vi "reconnaissance couleur (SubVI).vi"(8 "error in (no error)":errorcluster, 9 "Image Out in":T2, 10 "ROI Descriptor (Color Classification 1)":T1, 11 "Refnum in":T3) -> (1 "Array":errorcluster[](array[cluster]), 2 "Array 2":string[](array[string]), 3 "Refnum out":T2)   [LabVIEW 2019]
uses:
  <vilib>/vision/Image Controls.llb/IMAQ Image.ctl
  <vilib>/vision/Classification.llb/IMAQ Classifier Session.ctl
  <vilib>/vision/NI_Vision_Development_Module.lvlib
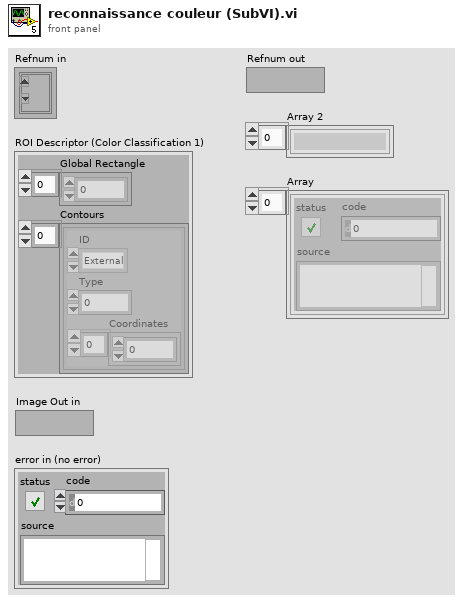
[diagram p1: front panel]
types:
  T1 = cluster{"Global Rectangle":i32[], "Contours":cluster{"ID":enum32{"External", "Internal"}, "Type":u32, "Coordinates":i32[]}[]}
  T2 = typedef "IMAQ Image.ctl" = refnum<image>
  T3 = typedef "IMAQ Classifier Session.ctl" = refnum<k1>
  T4 = typedef "ROI Descriptor" = cluster{"Global Rectangle":i32[], "Contours":cluster{"ID":enum32{"External", "Internal"}, "Type":u32, "Coordinates":i32[]}[]}
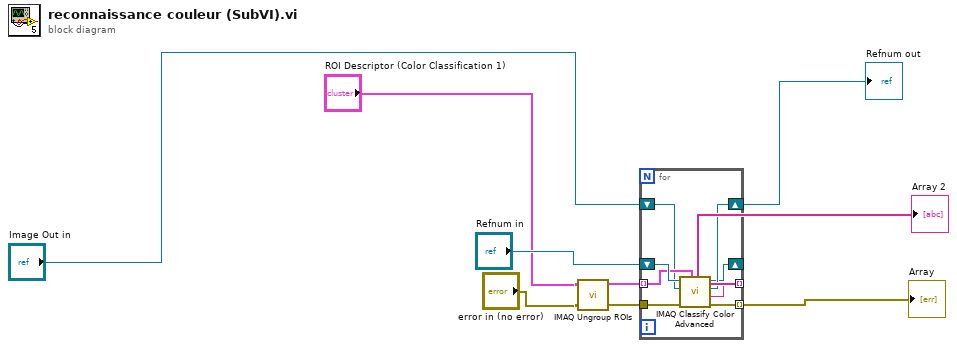
[diagram p0: block diagram]
diagram:
  n1 = call "IMAQ Ungroup ROIs"("error in (no error)"="error in (no error)", "ROI Descriptor"="ROI Descriptor (Color Classification 1)") -> ("error out"=w4:errorcluster, "ROI Descriptors out"=w5:T4[])  [unwired: 2 out]
  n2 = for {
    tunnel: [w17] -> w1 mode=indexing
    tunnel: [w16] -> w6 mode=indexing
    tunnel: w4 -> [w14]
    tunnel: w5 -> [w13] mode=indexing
    shift-right: [w11] -> w9
    shift-left: "Image Out in" -> [w12]
    shift-right: [w10] -> _
    shift-left: "Refnum in" -> [w15]
    n3 = call "IMAQ Classify Color Advanced"("ROI Descriptor"=w13, "error in (no error)"=w14, "Image"=w12, "Classifier Session"=w15) -> ("error out"=w16:errorcluster, "Class"=w17:string, "Image (dup)"=w11:T2, "Classifier Session (dup)"=w10:T3)  [unwired: 4 out]
  }
  "Refnum out" <- w9
  "Array" <- w6
  "Array 2" <- w1
